vi "PathPlanner_PathPoint_GetAll.vi"(11 "PathPlannerPoint":T4={"Position"={"X"=0.0, "Y"=0.0}, "HolonomicRotation"={"VALUE"=0.0, "COS"=1.0, "SIN"=0.0}, "DistAlongPath"=0.0, "CurveRadius"=0.0, "MaxV"=9e+300, "Constraints"={"MaxVelocityMps;"=0.0, "MaxAccelerationMpsSq;"=0.0, "MaxAngularVelRadPsEc;"=0.0, "MaxAngularAccRadPSecSq"=0.0, "Exists"=FALSE}, "HolonomicRotationExists"=FALSE} {"HolonomicRotation"."SIN" format="%13.4f"; "HolonomicRotation"."COS" format="%13.4f"; "HolonomicRotation"."VALUE" format="%13.4f"; "Position"."Y" format="%14.3f"; "Position"."X" format="%14.3f"}) -> (0 "DistAlongPath":dbl, 1 "Constraints":T1, 2 "HolonomicRotation":T2={"VALUE"=0.0, "COS"=1.0, "SIN"=0.0} {"SIN" format="%13.4f"; "COS" format="%13.4f"; "VALUE" format="%13.4f"}, 3 "Position":T3 {"Y" format="%14.3f"; "X" format="%14.3f"}, 4 "CurveRadius":dbl, 6 "MaxV":dbl, 8 "HolonomicRotationExists":bool)   [LabVIEW 2019, in "PathPlanner24.lvlib"]
doc: "/**\n * Create a new path constraints object\n *\n * @param maxVelocityMps Max linear velocity (M/S)\n * @param maxAccelerationMpsSq Max linear acceleration (M/S^2)\n * @param maxAngularVelocityRps Max angular velocity (Rad/S)\n * @param maxAngularAccelerationRpsSq Max angular acceleration (Rad/S^2)\n */"
uses:
  PathPlanner24.lvlib
  TypeDef/PathPlannerPathPoint.ctl
  <vilib>/Rock Robotics/WPI/ThirdParty/JAS_Junk/TrajLib/TypeDef/TRANSLATION2D.ctl
  <vilib>/Rock Robotics/WPI/ThirdParty/JAS_Junk/TrajLib/TypeDef/ROTATION2D.ctl
  TypeDef/PathPlannerPathConstraints.ctl
  <vilib>/Rock Robotics/WPI/ThirdParty/JAS_Junk/TrajLib/Trajectory_Library.lvlib
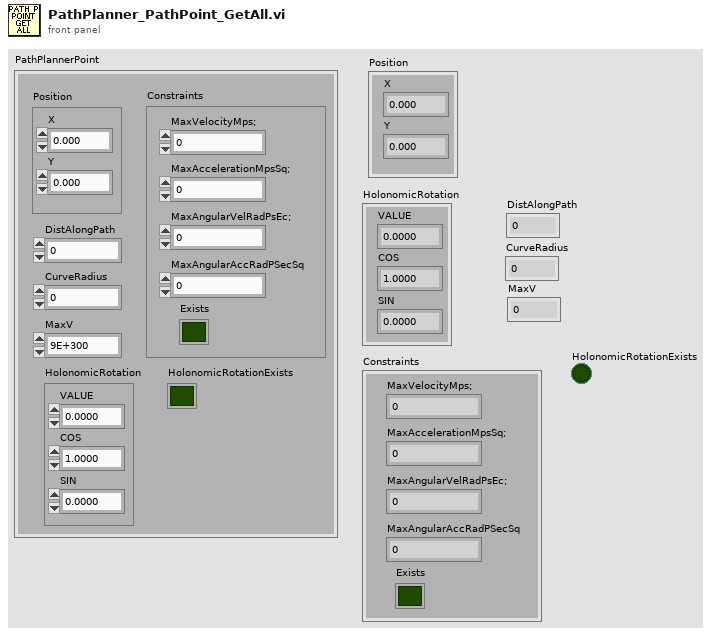
[diagram p1: front panel]
types:
  T1 = typedef "PathPlanner24.lvlib/PathPlannerPathConstraints.ctl" = cluster{"MaxVelocityMps;":dbl, "MaxAccelerationMpsSq;":dbl, "MaxAngularVelRadPsEc;":dbl, "MaxAngularAccRadPSecSq":dbl, "Exists":bool}
  T2 = typedef "Trajectory_Library.lvlib/ROTATION2D.ctl" = cluster{"VALUE":dbl, "COS":dbl, "SIN":dbl}
  T3 = typedef "Trajectory_Library.lvlib/TRANSLATION2D.ctl" = cluster{"X":dbl, "Y":dbl}
  T4 = typedef "PathPlanner24.lvlib/PathPlannerPathPoint.ctl" = cluster{"Position":T3, "HolonomicRotation":T2, "DistAlongPath":dbl, "CurveRadius":dbl, "MaxV":dbl, "Constraints":T1, "HolonomicRotationExists":bool}
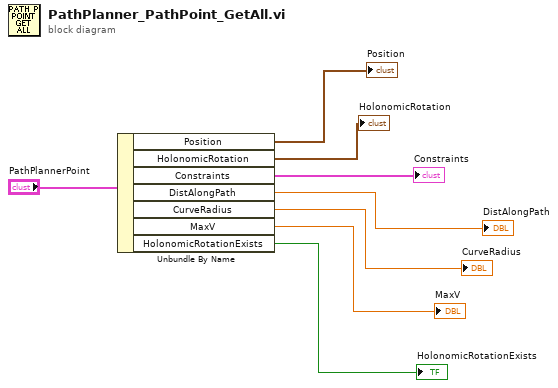
[diagram p0: block diagram]
diagram:
  n1 = Unbundle By Name("PathPlannerPoint") -> ("Position"=→"Position":T3, "HolonomicRotation"=→"HolonomicRotation":T2, "Constraints"=→"Constraints":T1, "DistAlongPath"=→"DistAlongPath":dbl, "CurveRadius"=→"CurveRadius":dbl, "MaxV"=→"MaxV":dbl, "HolonomicRotationExists"=→"HolonomicRotationExists":bool)
